vi "SetImageType.vi"(8 "error in (no error)":errorcluster, 10 "Image Type":u8 format="%.0x", 11 "CameraTesting in":refnum<class "CameraTesting.lvclass">) -> (0 "error out":errorcluster, 3 "CameraTesting out":refnum<class "CameraTesting.lvclass">)   [LabVIEW 2020, in "CameraTesting.lvlib" / "CameraTesting.lvclass"]
uses:
  CameraTesting.lvclass
  CameraTesting.lvclass/CameraTesting.ctl
  Camera/ICamera/ICamera/ICamera.lvclass
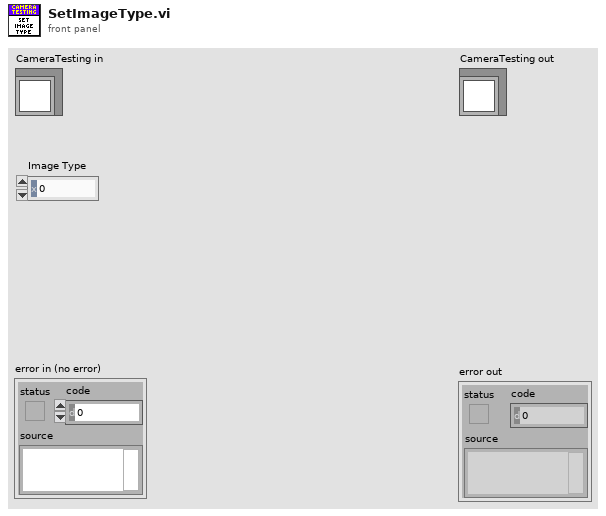
[diagram p1: front panel]
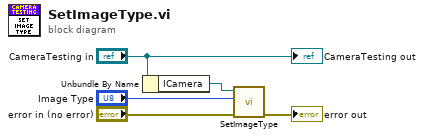
[diagram p0: block diagram]
diagram:
  n1 = Unbundle By Name("CameraTesting in") -> ("ICamera"=w3:refnum<class "ICamera.lvclass">)
  n2 = call-dynamic "SetImageType.vi"("error in (no error)"="error in (no error)", "Image Type (hex code)"="Image Type", "ICamera in"=w3) -> ("error out"=→"error out":errorcluster)  [unwired: 7 in, 1 out]
  "CameraTesting out" <- "CameraTesting in"
